vi "Periodic Tasks.vi"(0 "error in":errorcluster) -> ()   [LabVIEW 2019]
doc: "This VI runs in parallel to other tasks. It can contain as many user-defined periodic loops as you need. These can carry out PID or other sorts of timed response."
uses:
  dsinstructions.vi
  sensors.vi
  dsdata.vi
  constants.vi
  robotmodes.vi
  refnums.vi
  outputs.vi
panel:
  in  "Plot":bool
  out "PID Tracking":cluster{"Goal Wheel Position":dbl, dbl}(graph)={"Goal Wheel Position"=0.0, -90.17571233858979}
  out "Contribution Tracking":cluster{dbl, dbl, dbl}(graph)
  in  "Swerve N-Int":i32=10 caption="N-Int"
  in  "Swerve N-Diff":i32=10 caption="N-Diff"
  in  "Swerve Kd":dbl
  in  "Swerve Ki":dbl
  in  "Swerve Kp":dbl=0.005
  out "Drive Sequencer":i32
  out "Subsystem Action":path
  out "Time Since Latch (ms)":u32
  out "Subsystem Sequencer":i32
  out "Drive Action":string
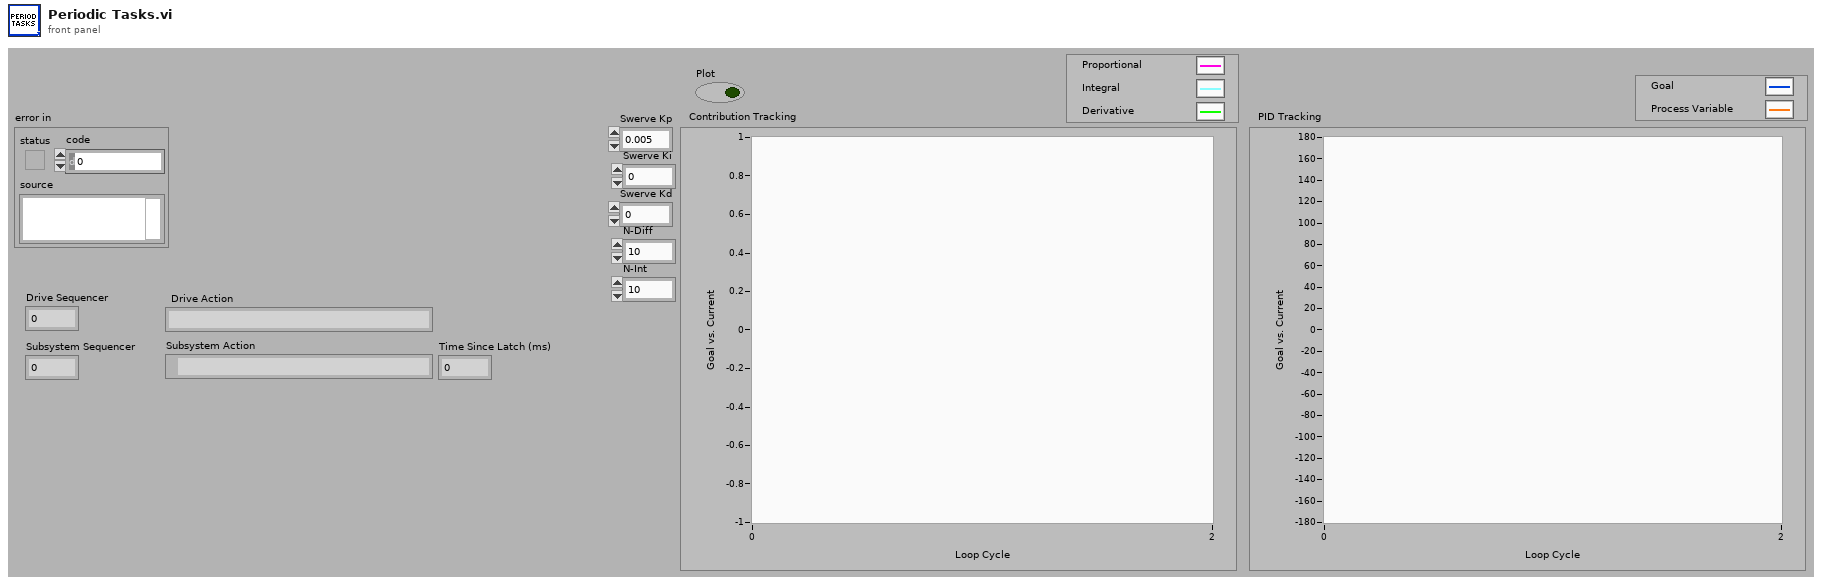
[diagram p1: front panel]
types:
  T1 = typedef "WPI_MotorControlDeviceRef.ctl" = cluster{"DeviceStatus":errorcluster, "Type":T2, "PWM":cluster{"PWM Channel":T3, "DeadBand":T4}, "CAN":cluster{"Device Number":u8, "SetOutput VI Ref":variant, "GetOutput VI Ref":variant, "Enable VI Ref":variant, "Disable VI Ref":variant, "Data":variant}, "Invert":bool, "DIO PWM":cluster{"PWM \"Enable\" Channel":T3, "DIOChannel":T5, "PWM Rate":dbl}}
  T2 = typedef "WPI_MotorControlType.ctl" = enum16{"PWM", "CAN", "DIO PWM"}
  T3 = typedef "FPGA_DIOPWMChannel.ctl" = enum8{"PWM 0", "PWM 1", "PWM 2", "PWM 3", "PWM 4", "PWM 5", "PWM 6", "PWM 7", "PWM 8", "PWM 9", "PWM MXP 0", "PWM MXP 1", "PWM MXP 2", "PWM MXP 3", "PWM MXP 4", "PWM MXP 5", "PWM MXP 6", "PWM MXP 7", "PWM MXP 8", "PWM MXP 9", "Invalid"}
  T4 = typedef "WPI_PWMDeadband.ctl" = cluster{"Name":string, "maxPositivePwm":i32, "minPositivePwm":i32, "centerPwm":i32, "maxNegativePwm":i32, "minNegativePwm":i32, "angularRange":u16}
  T5 = typedef "FPGA_DIOChannel.ctl" = enum8{"DIO 0", "DIO 1", "DIO 2", "DIO 3", "DIO 4", "DIO 5", "DIO 6", "DIO 7", "DIO 8", "DIO 9", "DIO MXP 0", "DIO MXP 1", "DIO MXP 2", "DIO MXP 3", "DIO MXP 4", "DIO MXP 5", "DIO MXP 6", "DIO MXP 7", "DIO MXP 8", "DIO MXP 9", "DIO MXP 10", "DIO MXP 11", "DIO MXP 12", "DIO MXP 13", "DIO MXP 14", "DIO MXP 15", "SPI Port CS1", "SPI Port CS2", "SPI Port CS3", "SPI Port MISO", "SPI Port MOSI", "Invalid"}
  T6 = typedef "WPI_DriverStationRobotMode2.ctl" = enum16{"Autonomous Disabled", "Autonomous Enabled", "Teleop Disabled", "Teleop Enabled", "Disconnected", "Finish", "Test Disabled", "Test Enabled", "Emergency Stopped"}
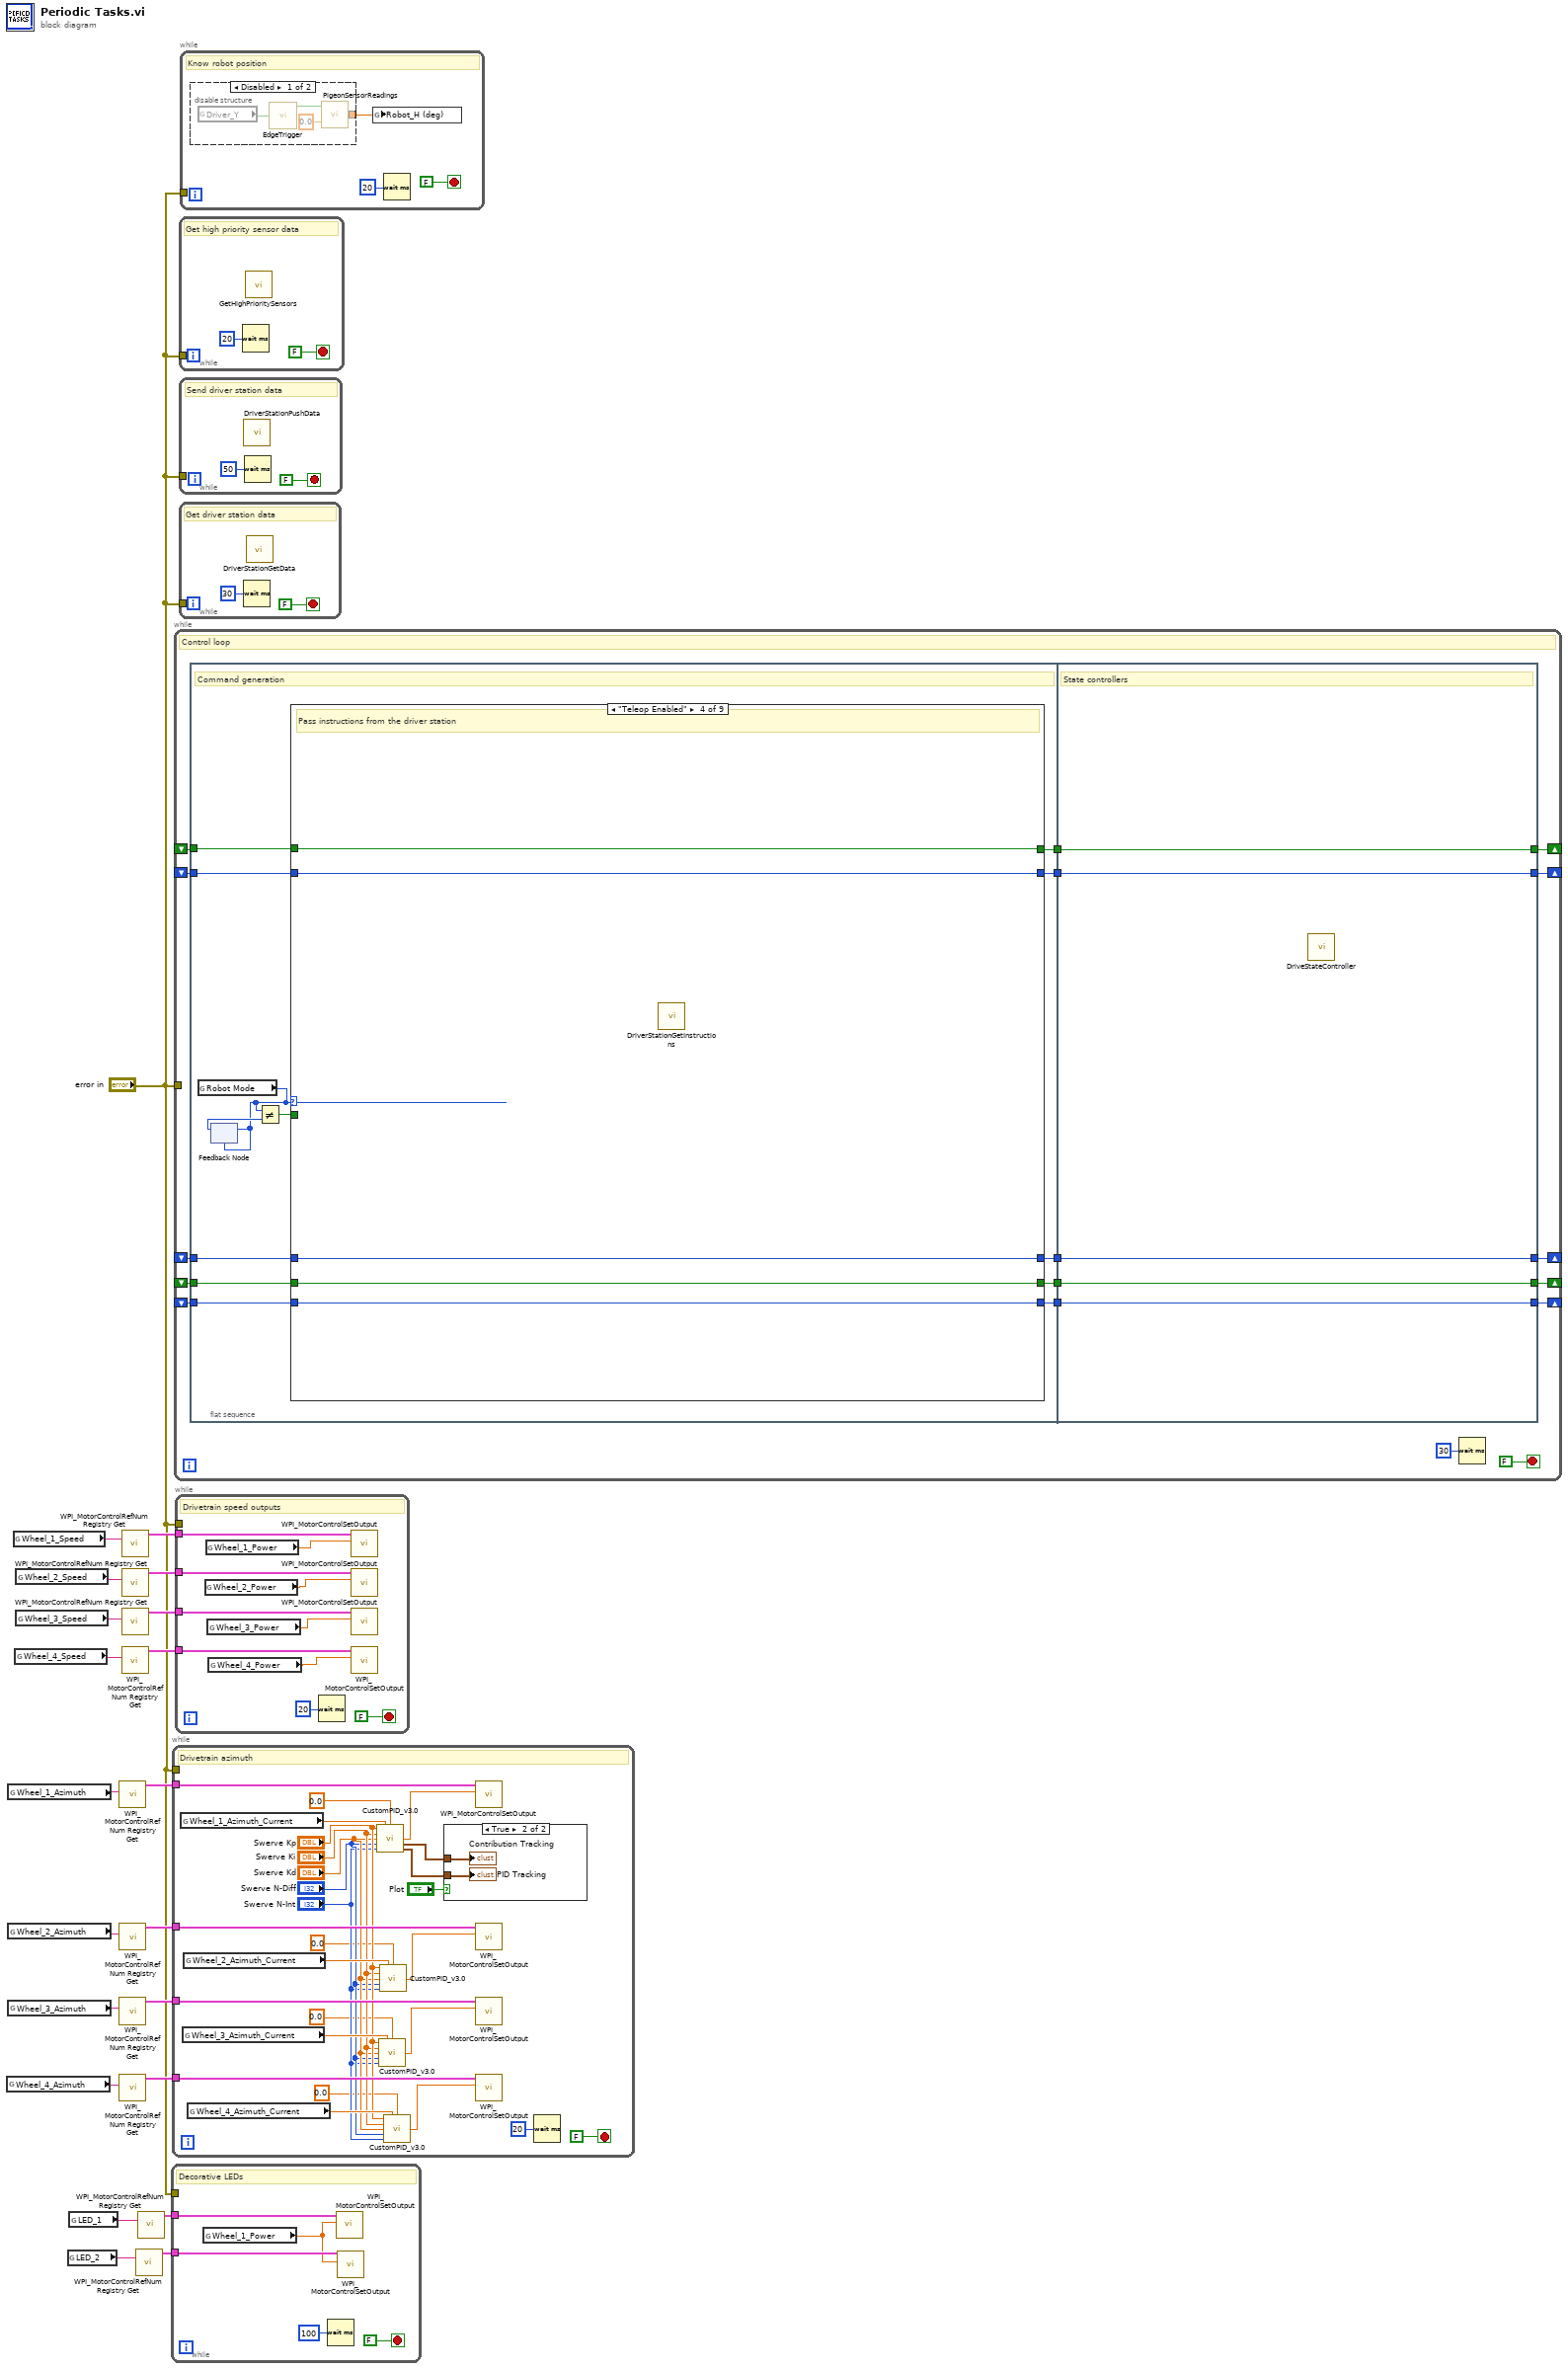
[diagram p0: block diagram]
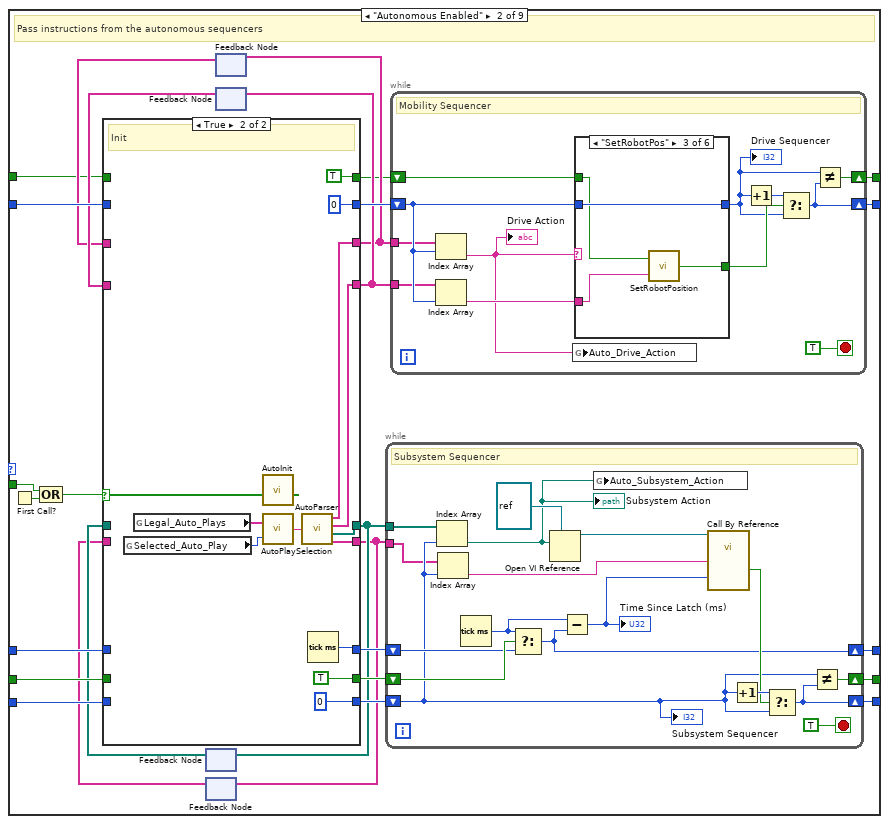
[diagram p5: hidden frame]
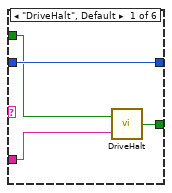
[diagram p6: hidden frame]
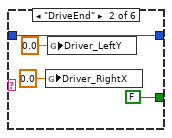
[diagram p7: hidden frame]
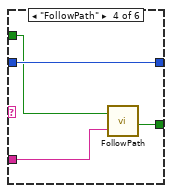
[diagram p8: hidden frame]
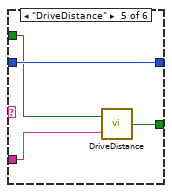
[diagram p9: hidden frame]
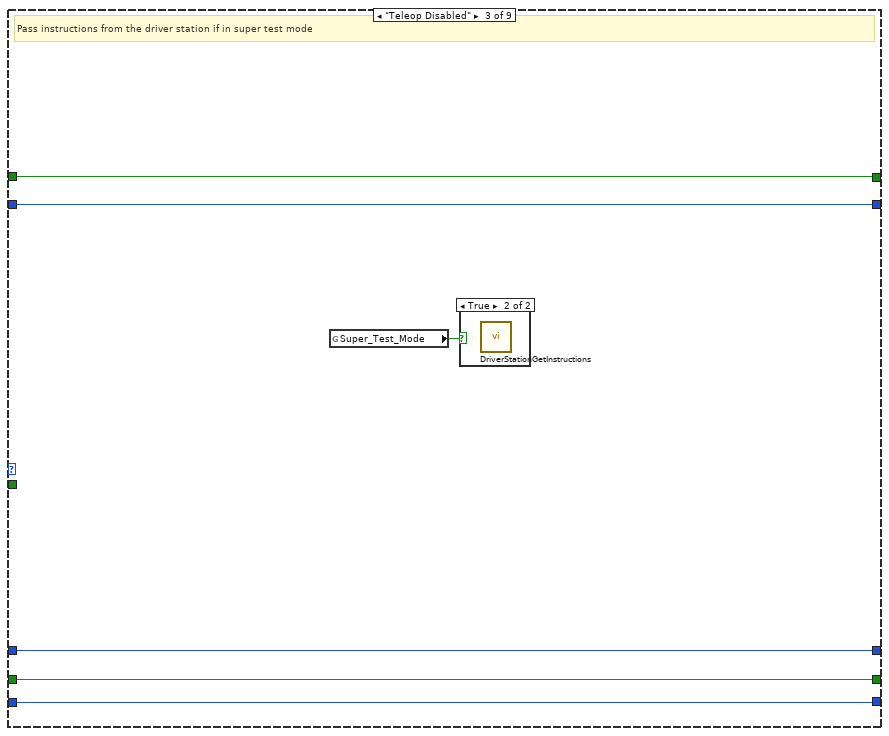
[diagram p12: hidden frame]
diagram:
  n1 = global read "refnums.vi" "Wheel_4_Azimuth"() -> (w6:string)
  n2 = global read "refnums.vi" "Wheel_1_Azimuth"() -> (w9:string)
  n3 = global read "refnums.vi" "Wheel_2_Azimuth"() -> (w8:string)
  n4 = global read "refnums.vi" "Wheel_3_Azimuth"() -> (w7:string)
  n5 = global read "refnums.vi" "Wheel_1_Speed"() -> (w17:string)
  n6 = global read "refnums.vi" "Wheel_4_Speed"() -> (w14:string)
  n7 = global read "refnums.vi" "Wheel_2_Speed"() -> (w16:string)
  n8 = global read "refnums.vi" "Wheel_3_Speed"() -> (w15:string)
  n9 = global read "refnums.vi" "LED_2"() -> (w2:string)
  n10 = global read "refnums.vi" "LED_1"() -> (w3:string)
  n11 = call <vilib>:"WPI_MotorControlRefNum Registry Get.vi"("refnum name"=w9) -> ("MotorControlDevRef"=w13:T1)  [unwired: 9 in, 1 out]
  n12 = call <vilib>:"WPI_MotorControlRefNum Registry Get.vi"("refnum name"=w8) -> ("MotorControlDevRef"=w12:T1)  [unwired: 9 in, 1 out]
  n13 = call <vilib>:"WPI_MotorControlRefNum Registry Get.vi"("refnum name"=w7) -> ("MotorControlDevRef"=w11:T1)  [unwired: 9 in, 1 out]
  n14 = call <vilib>:"WPI_MotorControlRefNum Registry Get.vi"("refnum name"=w6) -> ("MotorControlDevRef"=w10:T1)  [unwired: 9 in, 1 out]
  n15 = call <vilib>:"WPI_MotorControlRefNum Registry Get.vi"("refnum name"=w17) -> ("MotorControlDevRef"=w21:T1)  [unwired: 9 in, 1 out]
  n16 = call <vilib>:"WPI_MotorControlRefNum Registry Get.vi"("refnum name"=w16) -> ("MotorControlDevRef"=w20:T1)  [unwired: 9 in, 1 out]
  n17 = call <vilib>:"WPI_MotorControlRefNum Registry Get.vi"("refnum name"=w15) -> ("MotorControlDevRef"=w19:T1)  [unwired: 9 in, 1 out]
  n18 = call <vilib>:"WPI_MotorControlRefNum Registry Get.vi"("refnum name"=w14) -> ("MotorControlDevRef"=w18:T1)  [unwired: 9 in, 1 out]
  n19 = call <vilib>:"WPI_MotorControlRefNum Registry Get.vi"("refnum name"=w2) -> ("MotorControlDevRef"=w1:T1)  [unwired: 9 in, 1 out]
  n20 = call <vilib>:"WPI_MotorControlRefNum Registry Get.vi"("refnum name"=w3) -> ("MotorControlDevRef"=w4:T1)  [unwired: 9 in, 1 out]
  n21 = while {
    tunnel: "error in" -> [_]
    tunnel: w4 -> [w24]
    tunnel: w1 -> [w23]
    stop <- FALSE stop-if-true
    # "Decorative LEDs"
    n22 = global read "outputs.vi" "Wheel_1_Power"() -> (w22:dbl)
    n23 = Wait (ms)(milliseconds to wait=u32 100) -> ()  [unwired: 1 out]
    n24 = call <vilib>:"WPI_MotorControlSetOutput.vi"("Output"=w22, "MotorControlDevRef"=w24) -> ()  [unwired: 7 in, 3 out]
    n25 = call <vilib>:"WPI_MotorControlSetOutput.vi"("Output"=w22, "MotorControlDevRef"=w23) -> ()  [unwired: 7 in, 3 out]
  }
  n26 = while {
    tunnel: w13 -> [w50]
    tunnel: w12 -> [w49]
    tunnel: w11 -> [w48]
    tunnel: w10 -> [w47]
    tunnel: "error in" -> [_]
    stop <- FALSE stop-if-true
    # "Drivetrain azimuth"
    n27 = global read "outputs.vi" "Wheel_1_Azimuth_Current"() -> (w41:dbl)
    n28 = global read "outputs.vi" "Wheel_3_Azimuth_Current"() -> (w45:dbl)
    n29 = global read "outputs.vi" "Wheel_2_Azimuth_Current"() -> (w43:dbl)
    n30 = global read "outputs.vi" "Wheel_4_Azimuth_Current"() -> (w46:dbl)
    n31 = call "CustomPID_v3.0.vi"("Kp"="Swerve Kp", "Process Variable"=w41, "Goal"=0.0, "Ki"="Swerve Ki", "Kd"="Swerve Kd", "N-Diff"="Swerve N-Diff", "N-Int"="Swerve N-Int") -> ("Command"=w40:dbl, "Contribution Tracking"=w33:cluster{dbl, dbl, dbl}, "PID Tracking"=w32:cluster{"Goal Wheel Position":dbl, dbl})  [unwired: 5 in, 1 out]
    n32 = call "CustomPID_v3.0.vi"("Kp"="Swerve Kp", "Process Variable"=w45, "Goal"=0.0, "Ki"="Swerve Ki", "Kd"="Swerve Kd", "N-Diff"="Swerve N-Diff", "N-Int"="Swerve N-Int") -> ("Command"=w28:dbl)  [unwired: 5 in, 3 out]
    n33 = call "CustomPID_v3.0.vi"("Kp"="Swerve Kp", "Process Variable"=w43, "Goal"=0.0, "Ki"="Swerve Ki", "Kd"="Swerve Kd", "N-Diff"="Swerve N-Diff", "N-Int"="Swerve N-Int") -> ("Command"=w42:dbl)  [unwired: 5 in, 3 out]
    n34 = call "CustomPID_v3.0.vi"("Kp"="Swerve Kp", "Process Variable"=w46, "Goal"=0.0, "Ki"="Swerve Ki", "Kd"="Swerve Kd", "N-Diff"="Swerve N-Diff", "N-Int"="Swerve N-Int") -> ("Command"=w44:dbl)  [unwired: 5 in, 3 out]
    n35 = case shown="True" "Plot" {
      tunnel: w33 -> [_ w54]
      tunnel: w32 -> [_ w53]
      frame False {
      }
      frame True {
        "Contribution Tracking" <- w54
        "PID Tracking" <- w53
      }
    }
    n36 = call <vilib>:"WPI_MotorControlSetOutput.vi"("Output"=w40, "MotorControlDevRef"=w50) -> ()  [unwired: 7 in, 3 out]
    n37 = call <vilib>:"WPI_MotorControlSetOutput.vi"("Output"=w42, "MotorControlDevRef"=w49) -> ()  [unwired: 7 in, 3 out]
    n38 = call <vilib>:"WPI_MotorControlSetOutput.vi"("Output"=w28, "MotorControlDevRef"=w48) -> ()  [unwired: 7 in, 3 out]
    n39 = call <vilib>:"WPI_MotorControlSetOutput.vi"("Output"=w44, "MotorControlDevRef"=w47) -> ()  [unwired: 7 in, 3 out]
    n40 = Wait (ms)(milliseconds to wait=u32 20) -> ()  [unwired: 1 out]
  }
  n41 = while {
    tunnel: "error in" -> [_]
    shift-right: [w61] -> _
    shift-left: _ -> [w67]
    shift-right: [w62] -> _
    shift-left: _ -> [w68]
    shift-right: [w63] -> _
    shift-left: _ -> [w69]
    shift-right: [w59] -> _
    shift-left: _ -> [w58]
    shift-right: [w56] -> _
    shift-left: _ -> [w55]
    stop <- FALSE stop-if-true
    # "Control loop"
    n42 = flat-sequence {
      tunnel: w69 -> [w81]
      tunnel: w68 -> [w80]
      tunnel: w67 -> [w79]
      tunnel: [w84] -> w66
      tunnel: [w83] -> w65
      tunnel: [w82] -> w64
      tunnel: [w76] -> w60
      tunnel: w58 -> [w75]
      tunnel: [w74] -> w57
      tunnel: w55 -> [w73]
      tunnel: w66 -> [w227]
      tunnel: w65 -> [w226]
      tunnel: w64 -> [w225]
      tunnel: [w227] -> w63
      tunnel: [w226] -> w62
      tunnel: [w225] -> w61
      tunnel: w60 -> [w224]
      tunnel: [w224] -> w59
      tunnel: [w223] -> w56
      tunnel: w57 -> [w223]
      frame #0 {
        # "Command generation"
        n43 = global read "dsdata.vi" "Robot Mode"() -> (w72:T6)
        n44 = feedback-in #1(w72) -> ()
        n45 = feedback #1(w72) -> (w78:T6)
        n46 = Not Equal?(x=w72, y=w78) -> (x != y?=w77:bool)
        n47 = case shown="\"Teleop Enabled\"" w72 {
          tunnel: w81 -> [w89 w112 w190 w195 w200 w205 w210 w215 w220]
          tunnel: w80 -> [w88 w110 w189 w194 w199 w204 w209 w214 w219]
          tunnel: w79 -> [w87 w109 w188 w193 w198 w203 w208 w213 w218]
          tunnel: [w89 w115 w190 w195 w200 w205 w210 w215 w220] -> w84
          tunnel: [w88 w114 w189 w194 w199 w204 w209 w214 w219] -> w83
          tunnel: [w87 w113 w188 w193 w198 w203 w208 w213 w218] -> w82
          tunnel: w77 -> [_ w104 _ _ _ _ _ _ _]
          tunnel: [w86 w98 w191 w196 w201 w206 w211 w216 w221] -> w76
          tunnel: w75 -> [w86 w97 w191 w196 w201 w206 w211 w216 w221]
          tunnel: [w85 w91 w192 w197 w202 w207 w212 w217 w222] -> w74
          tunnel: w73 -> [w85 w90 w192 w197 w202 w207 w212 w217 w222]
          frame "Autonomous Disabled", Default {
          }
          frame "Autonomous Enabled" {
            # "Pass instructions from the autonomous sequencers"
            n48 = First Call?() -> (First Call?: T/F=w105:bool)
            n49 = Compound Arithmetic op=OR(w104, w105) -> (w106:bool)
            n50 = feedback #2() -> (w101:path[])  [unwired: 1 in]
            n51 = feedback #3() -> (w100:string[])  [unwired: 1 in]
            n52 = feedback #4() -> (w93:string[])  [unwired: 1 in]
            n53 = feedback #5() -> (w94:string[])  [unwired: 1 in]
            n54 = case shown="True" w106 {
              tunnel: w109 -> [w155 _]
              tunnel: w110 -> [w156 _]
              tunnel: w112 -> [w157 _]
              tunnel: [w157 w169] -> w111
              tunnel: [w156 TRUE ("Advance Trigger")] -> w108
              tunnel: [w155 0] -> w107
              tunnel: [w154 w162] -> w103
              tunnel: [w153 w166] -> w102
              tunnel: w101 -> [w154 _]
              tunnel: w100 -> [w153 _]
              tunnel: [w152 0] -> w99
              tunnel: w97 -> [w152 _]
              tunnel: [w151 w164] -> w96
              tunnel: [w150 w163] -> w95
              tunnel: w94 -> [w151 _]
              tunnel: w93 -> [w150 _]
              tunnel: [w149 TRUE] -> w92
              tunnel: w90 -> [w149 _]
              frame False {
                # "Pass"
              }
              frame True {
                # "Init"
                n55 = global read "dsdata.vi" "Selected_Auto_Play"() -> (w160:u16)
                n56 = global read "constants.vi" "Legal_Auto_Plays"() -> (w159:string[])
                n57 = call "AutoInit.vi"() -> ()  [unwired: 1 in]
                n58 = call "AutoPlaySelection.vi"("Selected Auto Play"=w160, "Auto Plays"=w159) -> ("Autonomous Commands"=w158:string)
                n59 = call "AutoParser.vi"("Auto Play"=w158) -> ("Drive Mode Strings"=w163:string[], "Drive Command Strings"=w164:string[], "Subsystem VI References"=w162:path[], "Subsystem Command Strings"=w166:string[])
                n60 = Tick Count (ms)() -> (millisecond timer value=w169:u32)
              }
            }
            n61 = feedback-in #2(w103) -> ()
            n62 = feedback-in #3(w102) -> ()
            n63 = feedback-in #4(w95) -> ()
            n64 = feedback-in #5(w96) -> ()
            n65 = while {
              tunnel: w103 -> [w174]
              shift-right: [w182] -> w113
              shift-left: w107 -> [w173]
              shift-right: [w181] -> w114
              shift-left: w108 -> [w180]
              shift-right: [w178] -> w115
              shift-left: w111 -> [w179]
              tunnel: w102 -> [w172]
              stop <- TRUE stop-if-true
              # "Subsystem Sequencer"
              n66 = Index Array(array=w174, index=w173) -> (element=w170:path)
              "Subsystem Action" <- w170
              n67 = Index Array(array=w172, index=w173) -> (element=w171:string)
              n68 = Tick Count (ms)() -> (millisecond timer value=w177:u32)
              n69 = Select(t=w177, s=w180, f=w179) -> (s? t:f=w178:u32)
              n70 = Open VI Reference(type specifier VI Refnum (for type only)=refnum<vi> refnum, vi path=w170) -> (vi reference=w176:refnum<vi>)  [unwired: 4 in, 1 out]
              n71 = Subtract(x=w177, y=w178) -> (x-y=w175:u32)
              "Time Since Latch (ms)" <- w175
              n72 = global write "robotmodes.vi" "Auto_Subsystem_Action"(w170) -> ()
              n73 = call-by-ref "?"(reference=w176, "Time Since Latch"=w175, "Instruction String"=w171) -> ("Advance Trigger"=w183:bool)  [unwired: 1 in, 2 out]
              n74 = Increment(x=w173) -> (x+1=w185:i32)
              n75 = Select(t=w185, s=w183, f=w173) -> (s? t:f=w182:i32)
              n76 = Not Equal?(x=w173, y=w182) -> (x != y?=w181:bool)
              "Subsystem Sequencer" <- w173
            }
            n77 = while {
              shift-right: [w120] -> w98
              shift-left: w99 -> [w125]
              tunnel: w95 -> [w124]
              tunnel: w96 -> [w123]
              shift-right: [w119] -> w91
              shift-left: w92 -> [w118]
              stop <- TRUE stop-if-true
              # "Mobility Sequencer"
              n78 = Index Array(array=w124, index=w125) -> (element=w116:string)
              "Drive Action" <- w116
              n79 = Index Array(array=w123, index=w125) -> (element=w122:string)
              n80 = global write "robotmodes.vi" "Auto_Drive_Action"(w116) -> ()
              n81 = case shown="\"SetRobotPos\"" w116 {
                tunnel: w125 -> [w131 w135 w139 w143 w147 w148]
                tunnel: [w131 w135 w139 w143 w147 w148] -> w117
                tunnel: w122 -> [w128 _ w137 w140 w145 _]
                tunnel: [w130 FALSE ("Increment") w138 w142 w144 _] -> w121
                tunnel: w118 -> [w129 _ w136 w141 w146 _]
                frame "DriveHalt", Default {
                  n82 = call "DriveHalt.vi"("Parameter String"=w128, "Reinit"=w129) -> ("Increment"=w130:bool)
                }
                frame "DriveEnd" {
                  n83 = global write "dsinstructions.vi" "Driver_RightX"(0.0 ("Driver_RightX")) -> ()
                  n84 = global write "dsinstructions.vi" "Driver_LeftY"(0.0 ("Driver_LeftY")) -> ()
                }
                frame "SetRobotPos" {
                  n85 = call "SetRobotPosition.vi"("Parameter String"=w137, "Reinit"=w136) -> ("Increment"=w138:bool)
                }
                frame "FollowPath" {
                  n86 = call "FollowPath.vi"("Parameter String"=w140, "Reinit"=w141) -> ("Increment"=w142:bool)
                }
                frame "DriveDistance" {
                  n87 = call "DriveDistance.vi"("Parameter String"=w145, "Reinit"=w146) -> ("Increment"=w144:bool)
                }
                frame "RotateAngle" {
                }
              }
              "Drive Sequencer" <- w117
              n88 = Increment(x=w117) -> (x+1=w126:i32)
              n89 = Select(t=w126, s=w121, f=w117) -> (s? t:f=w120:i32)
              n90 = Not Equal?(x=w117, y=w120) -> (x != y?=w119:bool)
            }
          }
          frame "Teleop Disabled" {
            # "Pass instructions from the driver station if in super test mode"
            n91 = global read "dsdata.vi" "Super_Test_Mode"() -> (w187:bool)
            n92 = case shown="True" w187 {
              frame False {
              }
              frame True {
                n93 = call "DriverStationGetInstructions.vi"() -> ()  [unwired: 12 in]
              }
            }
          }
          frame "Teleop Enabled" {
            # "Pass instructions from the driver station"
            n94 = call "DriverStationGetInstructions.vi"() -> ()  [unwired: 12 in]
          }
          frame "Finish" {
            # "Clean up operations are in the Finish.vi in RobotMain.vi"
          }
          frame "Test Disabled" {
            # "We are not using the testing mode"
          }
          frame "Test Enabled" {
            # "We are not using the testing mode"
          }
          frame "Disconnected" {
          }
          frame "Emergency Stopped" {
          }
        }
      }
      frame #1 {
        # "State controllers"
        n95 = call "DriveStateController.vi"() -> ()  [unwired: 1 in]
      }
    }
    n96 = Wait (ms)(milliseconds to wait=u32 30) -> ()  [unwired: 1 out]
  }
  n97 = while {
    tunnel: "error in" -> [_]
    tunnel: w21 -> [w235]
    tunnel: w20 -> [w234]
    tunnel: w19 -> [w233]
    tunnel: w18 -> [w232]
    stop <- FALSE stop-if-true
    # "Drivetrain speed outputs"
    n98 = global read "outputs.vi" "Wheel_2_Power"() -> (w230:dbl)
    n99 = global read "outputs.vi" "Wheel_1_Power"() -> (w231:dbl)
    n100 = global read "outputs.vi" "Wheel_3_Power"() -> (w228:dbl)
    n101 = global read "outputs.vi" "Wheel_4_Power"() -> (w229:dbl)
    n102 = Wait (ms)(milliseconds to wait=u32 20) -> ()  [unwired: 1 out]
    n103 = call <vilib>:"WPI_MotorControlSetOutput.vi"("Output"=w231, "MotorControlDevRef"=w235) -> ()  [unwired: 7 in, 3 out]
    n104 = call <vilib>:"WPI_MotorControlSetOutput.vi"("Output"=w230, "MotorControlDevRef"=w234) -> ()  [unwired: 7 in, 3 out]
    n105 = call <vilib>:"WPI_MotorControlSetOutput.vi"("Output"=w228, "MotorControlDevRef"=w233) -> ()  [unwired: 7 in, 3 out]
    n106 = call <vilib>:"WPI_MotorControlSetOutput.vi"("Output"=w229, "MotorControlDevRef"=w232) -> ()  [unwired: 7 in, 3 out]
  }
  n107 = while {
    tunnel: "error in" -> [_]
    stop <- FALSE stop-if-true
    # "Get high priority sensor data"
    n108 = Wait (ms)(milliseconds to wait=u32 20) -> ()  [unwired: 1 out]
    n109 = call "GetHighPrioritySensors.vi"() -> ()  [unwired: 1 in]
  }
  n110 = while {
    tunnel: "error in" -> [_]
    stop <- FALSE stop-if-true
    # "Get driver station data"
    n111 = Wait (ms)(milliseconds to wait=u32 30) -> ()  [unwired: 1 out]
    n112 = call "DriverStationGetData.vi"() -> ()  [unwired: 1 in]
  }
  n113 = while {
    tunnel: "error in" -> [_]
    stop <- FALSE stop-if-true
    # "Send driver station data"
    n114 = call "DriverStationPushData.vi"() -> ()  [unwired: 12 in]
    n115 = Wait (ms)(milliseconds to wait=u32 50) -> ()  [unwired: 1 out]
  }
  n116 = while {
    tunnel: "error in" -> [_]
    stop <- FALSE stop-if-true
    # "Know robot position"
    n117 = disable-structure shown="Disabled" {
      disable-tunnel: [w248 _] -> w244
      frame Disabled {
        n118 = global read "dsinstructions.vi" "Driver_Y"() -> (w249:bool)
        n119 = call "EdgeTrigger.vi"("Input Signal"=w249) -> ("Rising Edge Trigger"=w250:bool)  [unwired: 2 out]
        n120 = call "PigeonSensorReadings.vi"("Reset Yaw (deg)"=0.0, "Reset Yaw"=w250) -> ("Yaw (deg)"=w248:dbl)
      }
      frame Enabled {
      }
    }
    n121 = global write "sensors.vi" "Robot_H (deg)"(w244) -> ()
    n122 = Wait (ms)(milliseconds to wait=u32 20) -> ()  [unwired: 1 out]
  }
